vi "Update Waypoint Dictionary ConfigFile.vi"() -> ()   [LabVIEW 2020, in "WyPtDict.lvlib"]
uses:
  WyPtDict.lvlib
  RoboWaypointDict Node--cluster.ctl
  BRS_Dev/Source Code/Robo Driver/Controls/MC and Robo Handshake.ctl
  <vilib>/TELLC/Dynamic CVT API/TD Dynamic CVT DVR--ref.ctl
  <userlib>/_OpenG.lib/file/file.llb/File Exists - Scalar__ogtk.vi
panel:
  in  "Exit":bool
  in  "Save ConfigFile":bool
  in  "Load ConfigFile":bool
  in  "WyPtDictNode":T1[](array[typedef]) caption="Waypoint Configuration"
  in  "WaypointDictionary":T3
  in  "MainUI ViRef":refnum<vi>
  out "error out":errorcluster
  in  "error in (no error)":errorcluster
  out "Waypoint ConfigFile":path
  in  "WaypointDictionary":cluster{"WyPtDictNode":T1[]}
  # "XML Configuration File"
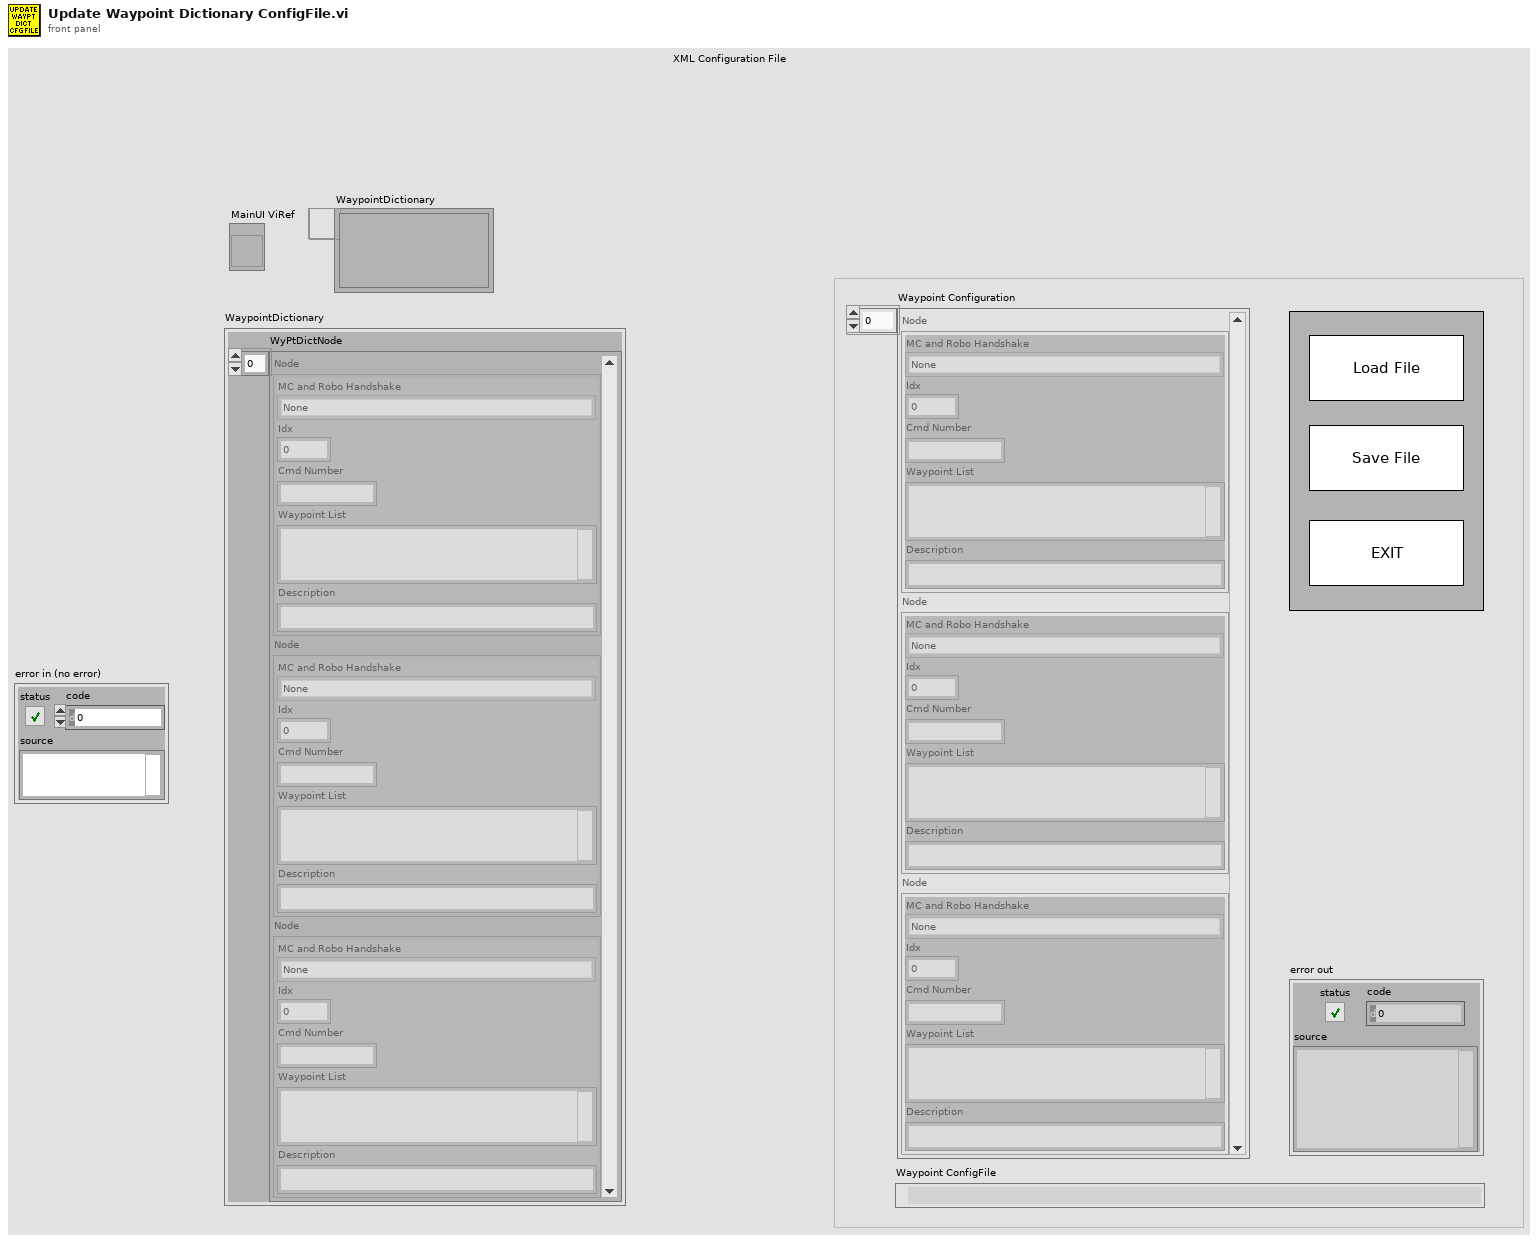
[diagram p1: front panel]
types:
  T1 = typedef "WyPtDict.lvlib/RoboWaypointDict Node--cluster.ctl" = cluster{"MC and Robo Handshake":T2, "Idx":i32, "Cmd Number":string, "Waypoint List":string, "Description":string}
  T2 = typedef "MC and Robo Handshake.ctl" = enum16{"None", "Move and Pick Nikon Ret LP(1100)", "Nikon Barcode1 Scanning Started(1101)", "Nikon Barcode1 Scan Abort(1102)", "Nikon Barcode1 Scan Success Proc to Barcode 2 Pos(1103)", "Nikon Barcode 2 Scanning Started(1104)", "Nikon Barcode 2 Scan Abort(1105) ", "Nikon Barcode 2 Success(1106)", "Move and Pick POZZ Ret LP(1300)", "POZZ Barcode Scan Started(1301)", "POZZ Barcode Not Found(1302)", "POZZ Barcode Scan Succ(1303)", "POZZ Mov to Side 2 Bar 2(1310)", "POZZ Mov to Side 4 Bar 1(1311)", "POZZ Mov to Side 4 Bar 2(1312)", "POZZ Mov to Side 1 Bar 1(1313)", "POZZ Mov to Side 1 Bar 2(1314)", "POZZ Mov to Side 3 Bar 1(1315)", "POZZ Mov to Side 3 Bar 2(1316)", "POZZ Mov to Edge 3 Nik 2(1317)", "POZZ Mov to Edge 4 ASML(1318)", "POZZ Mov to Edge 4 Nik 1(1319)", "POZZ Mov to Edge 4 Nik 2(1320)", "Move to ASML LP and Pick Ret(2000)", "ASML1 Barcode Scan Started(2001)", "ASML1 Barcode Not Found(2002)", "ASML1 Barcode Scan Succ(2003)", "Start Load Seq for Nikon LP(3000)", "Start Load Seq for POZZ LP(3200)", "Start Load Seq for ASML LP(3400)", "Start Align End Grip Place Func(4000)", "Start Align End grip Pick Func(4001)", "Start Align Center Grip Place Func(4002)", "Start Align Center grip Pick Func(4003)", "Start Move from home to Cleaner(5000)", "Start Move to Final Cleaner Loc(5001)", "Start Move from Cleaner loc to home(5002)", "Start Move from home to PDS for Inspect(6000) ", "PDS Inspect Finished(6001)", "PDS EMO Recovery(6002)", "Store in Stocker(7001)", "Store in Expansion Stocker(7401)", "Retrive from Center Stocker(8001)", "Retrive Mov to Nikon BC1 Scan Pos(8002)", "Retrive Nikon BC1not found(8003)", "Retrive Nikon BC1 Scan Succ(8004)", "Retrive Nikon BC2 not found(8005)", "Retrive Nikon BC2 scan Succ(8006)", "Retrive Mov to Edge 1 ASML(8202) ", "Retrive Mov to Edge 1 Nikon 1(8203)", "Retrive Mov to Edge 1 Nikon 2(8204)", "Retrive Mov to Edge 2 ASML(8205)", "Retrive Mov to Edge 2 Nikon 1(8206)", "Retrive Mov to Edge 2 Nikon 2(8207)", "Retrive Mov to Edge 3 ASML (8208)", "Retrive Mov to Edge 3 Nikon 1(8209)", "Retrive Mov to Edge 3 Nikon 2(8210)", "Retrive Mov to Edge 4 ASML (8211)", "Retrive Mov to Edge 4 Nikon 1 (8212)", "Retrive Mov to Edge 4 Nikon 2 (8213)", "Retrive BC Scan Abort (8214)", "Retrive BC Scan Successful (8215)", "Retrive Mov to ASML BC scan Pos (8402) ", "Retrive ASML BC not found(8403)", "Retrive ASML BC Scan Succ(8404)", "Expansion Retrive Seq (8601)", "Cen Stocker move from home to Transit Nest(9000)", "Cen Stocker move from Transit Nest to home(9200)", "Exp Stocker move from home to Transit Nest(9400)", "Exp Stocker move from Transit Nest to home(9600)", "Move to R1 Home (1000)", "Move to R2 Home (1000)", "Store Left Stocker (7401)", "Retrieve Left Stocker (8601)", "EMO Recovery Center (1002)", "EMO Recovery Right (1002)", "Center Robo Status (8888)", "Right Robo Status (8888)"}
  T3 = typedef "TD Dynamic CVT DVR--ref.ctl" = refnum<data-value>
  T4 = enum32{"Invalid", "Standard", "Closed", "Hidden", "Minimized", "Maximized"}
  T5 = cluster{"Core":cluster{"Current VI Reference":refnum<vi>, "Close Panel on Exit?":bool}, "WyPtDictNode":T1[], "ConfigFile":path}
  T6 = cluster{"Current VI Reference":refnum<vi>, "Close Panel on Exit?":bool}
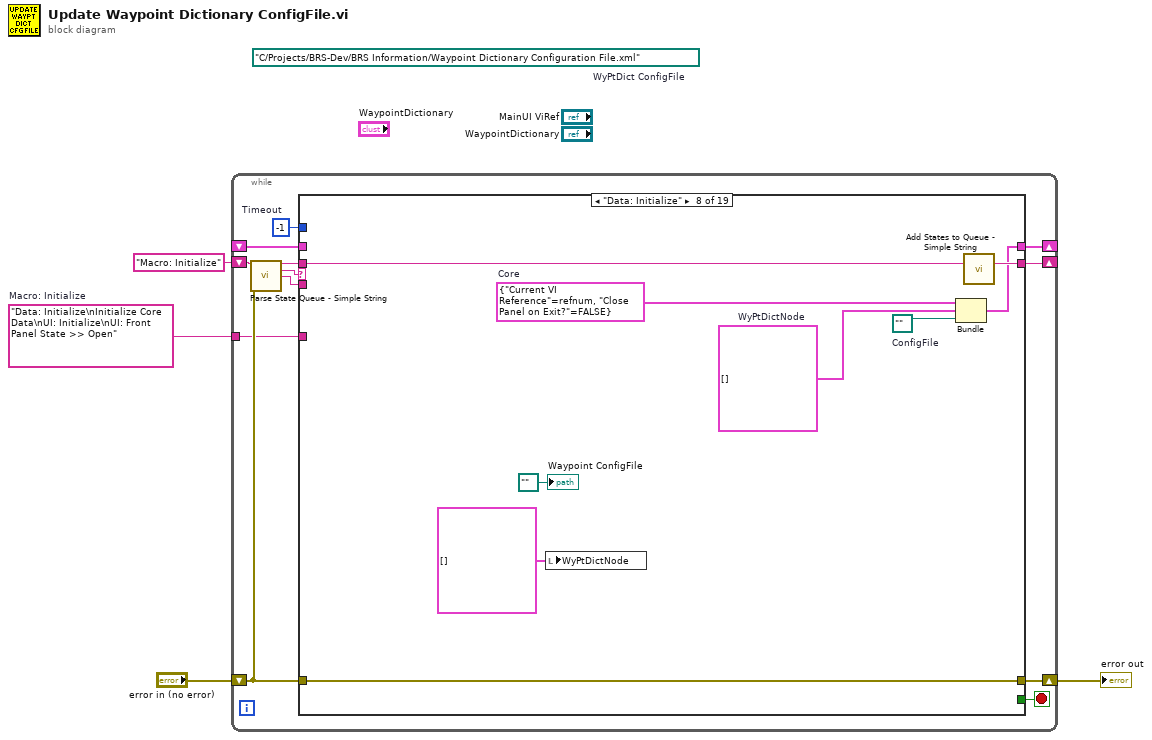
[diagram p0: block diagram]
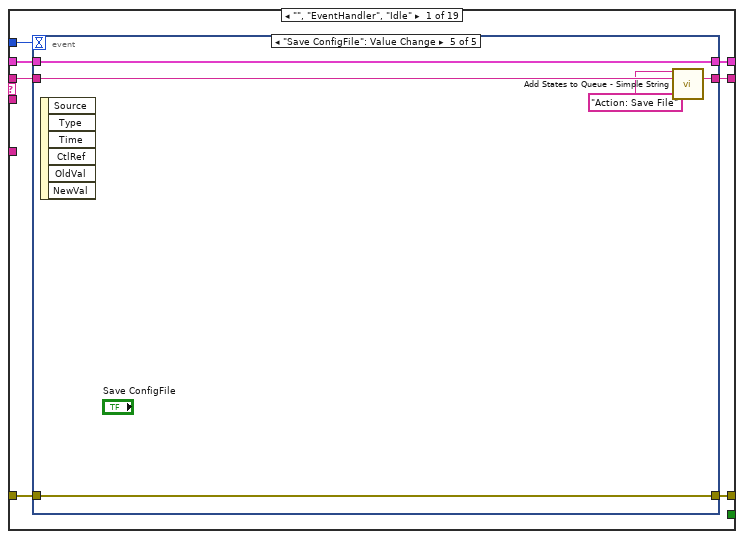
[diagram p2: hidden frame]
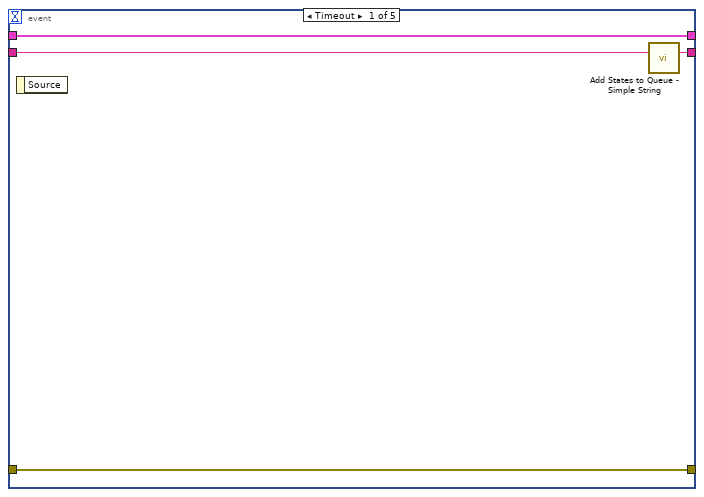
[diagram p3: hidden frame]
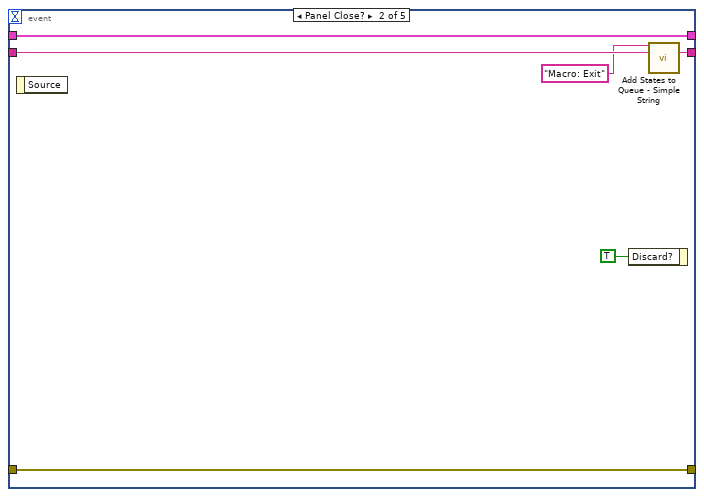
[diagram p4: hidden frame]
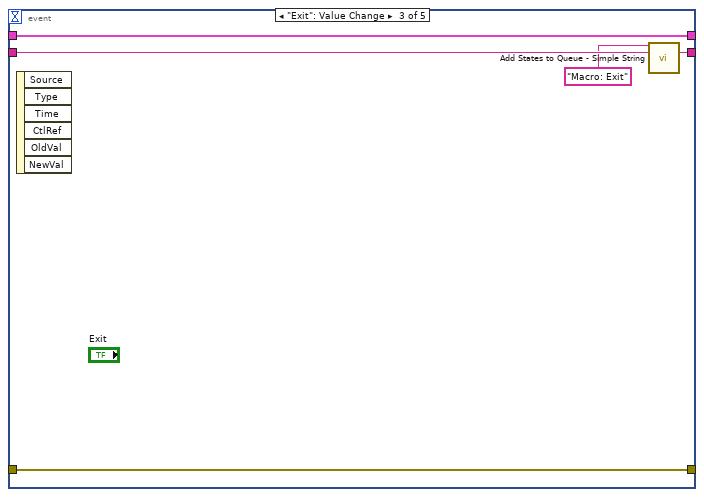
[diagram p5: hidden frame]
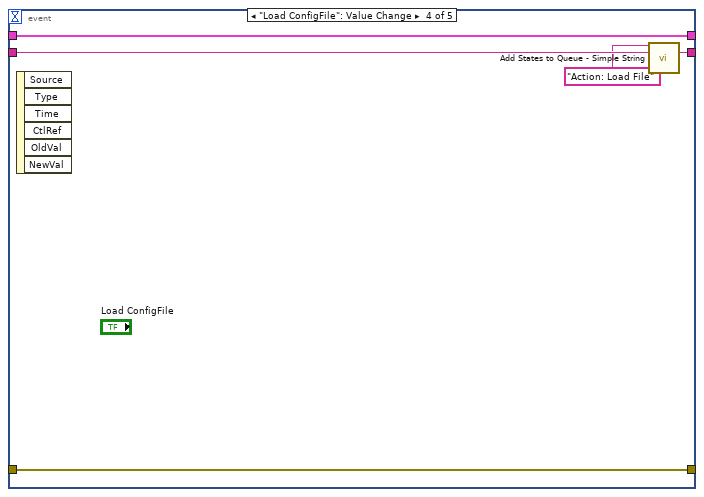
[diagram p6: hidden frame]
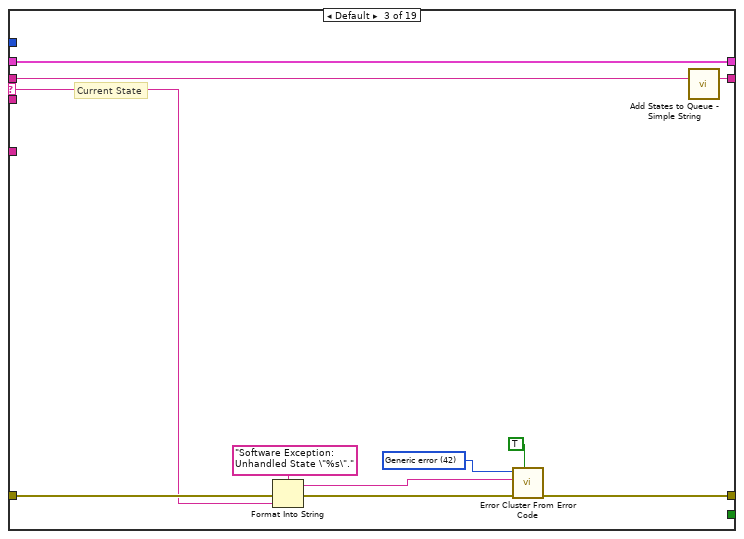
[diagram p8: hidden frame]
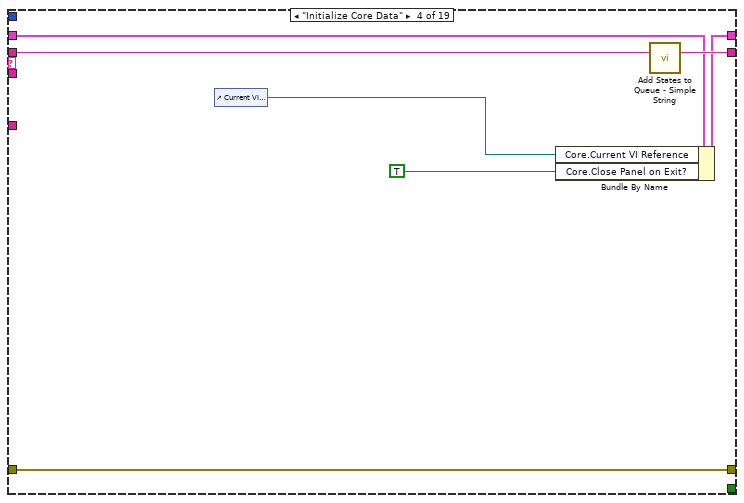
[diagram p9: hidden frame]
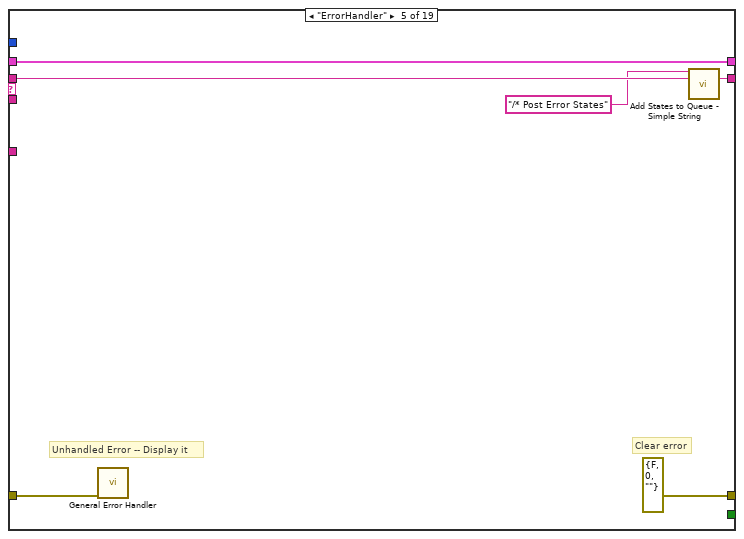
[diagram p10: hidden frame]
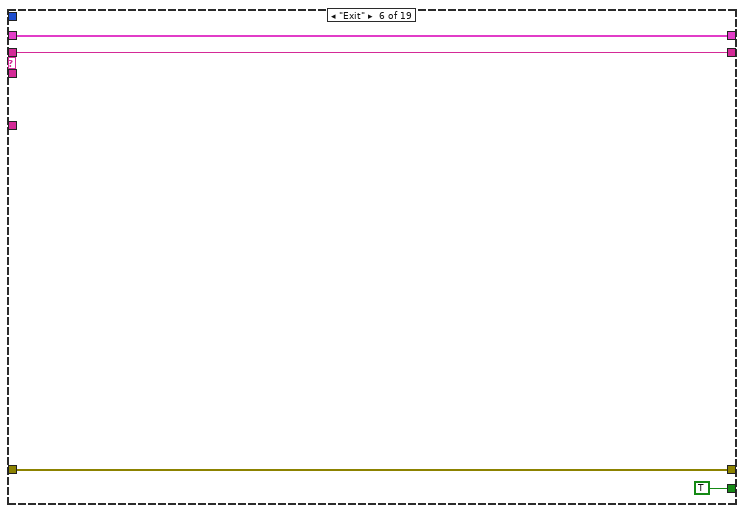
[diagram p11: hidden frame]
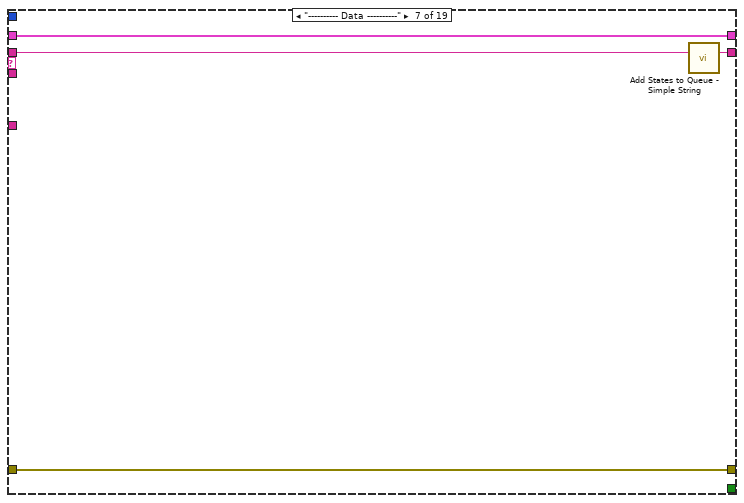
[diagram p12: hidden frame]
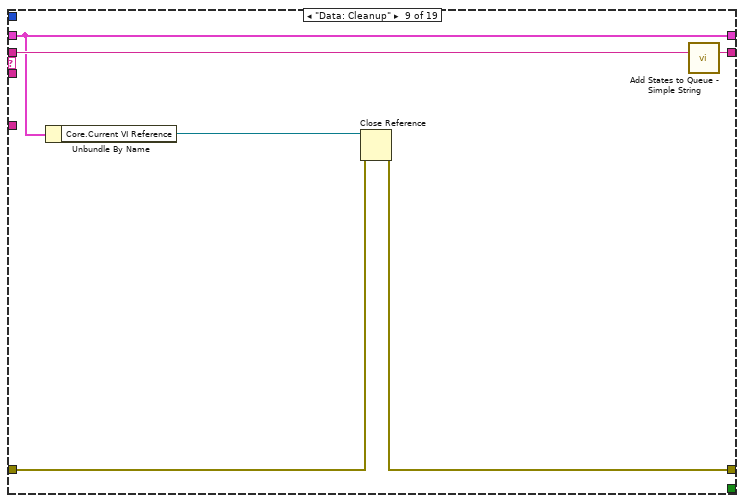
[diagram p13: hidden frame]
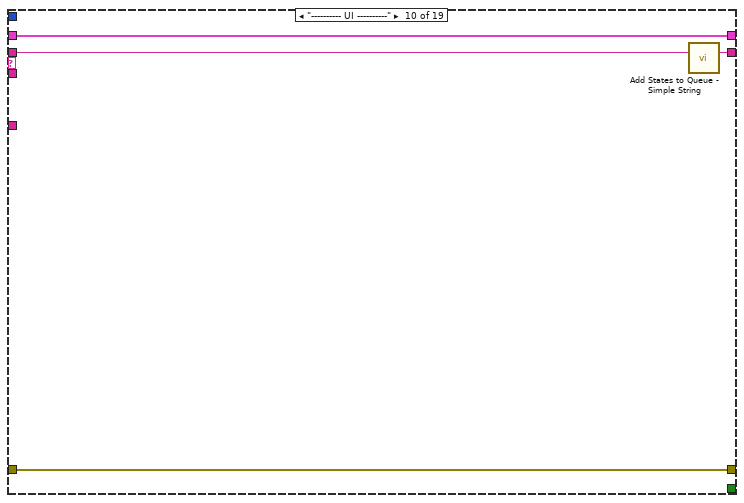
[diagram p14: hidden frame]
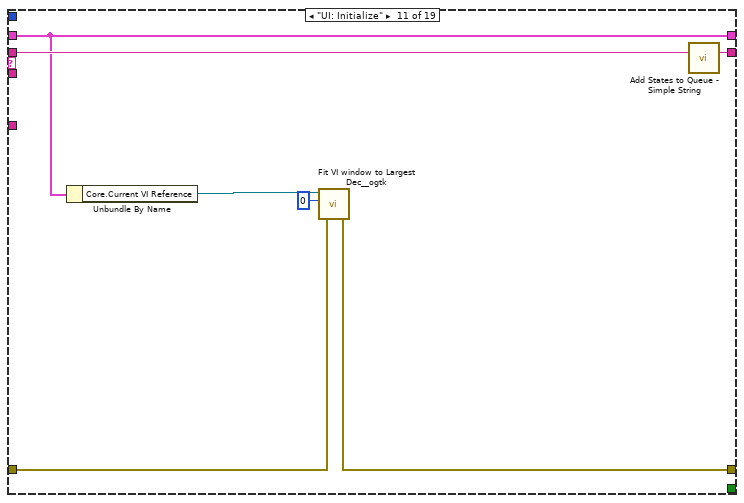
[diagram p15: hidden frame]
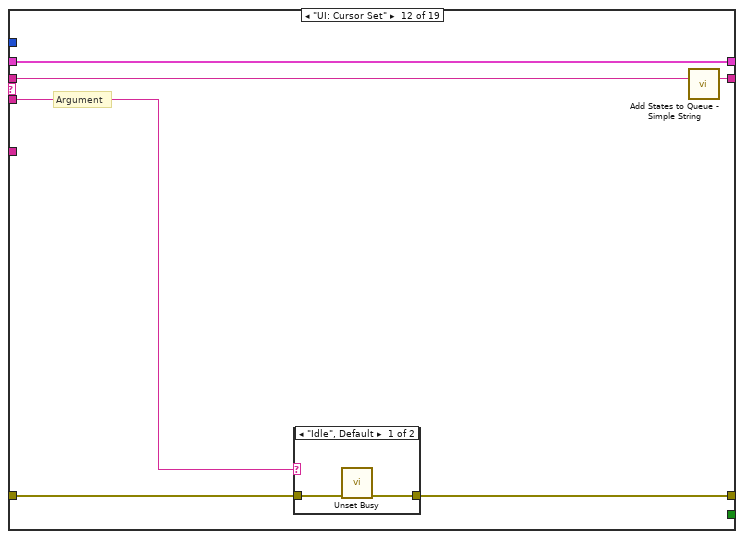
[diagram p16: hidden frame]
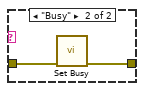
[diagram p17: hidden frame]
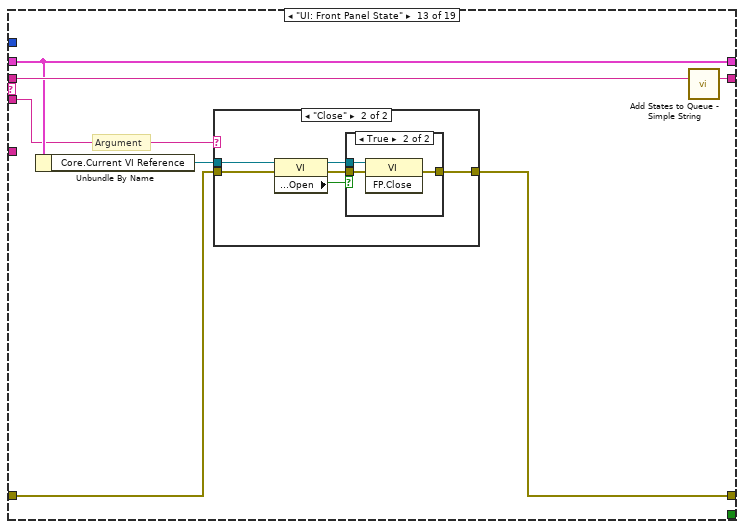
[diagram p18: hidden frame]
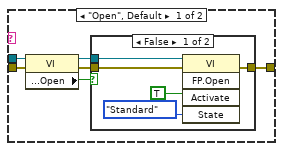
[diagram p19: hidden frame]
diagram:
  (unwired) path "C:/Projects/BRS-Dev/BRS Information/Waypoint Dictionary Configuration File.xml"  # WyPtDict ConfigFile
  w1 = "Data: Initialize\nInitialize Core Data\nUI: Initialize\nUI: Front Panel State >> Open"  # Macro: Initialize
  n1 = while {
    shift-right: [w9] -> _
    shift-left: _ -> [w8]
    shift-right: [w12] -> w3
    shift-left: "error in (no error)" -> [w6]
    shift-right: [w11] -> _
    shift-left: "Macro: Initialize" -> [w13]
    tunnel: w1 -> [w5]
    stop <- w10 stop-if-true
    w7 = -1  # Timeout
    n2 = call <vilib>:"Parse State Queue - Simple String.vi"("StateQ in"=w13, "error"=w6) -> ("Remaining States"=w15:string, "Next State"=w16:string, "Command (Optional)"=w14:string)  [unwired: 9 in, 2 out]
    n3 = case shown="\"Data: Initialize\"" w16 {
      selector: w16 -> [_ _ w52 _ _ _ _ _ _ _ _ _ _ _ _ _ _ _ _]
      tunnel: w15 -> [w23 w49 w56 w69 w75 w76 w83 w92 w98 w102 w109 w115 w126 w152 w157 w167 w171 w186 w208]
      tunnel: w14 -> [_ _ _ _ _ _ _ _ _ _ _ w110 w120 _ _ _ _ _ _]
      tunnel: w8 -> [w21 w50 w54 w65 w72 w79 w80 _ w93 w99 w107 w113 w122 w149 w154 w164 w168 w178 w203]
      tunnel: [w20 w51 w58 w66 errorcluster {"status"=FALSE, "code"=0, "source"=""} ("error out") w78 w81 w88 w94 w100 w104 w111 w123 w150 w155 w165 w169 w172 w199] -> w12
      tunnel: w6 -> [w19 w51 w57 w66 w71 w78 w81 w88 w95 w100 w103 w112 w124 w150 w155 w165 w169 w173 w200]
      tunnel: [w22 w49 w55 w68 w74 w76 w82 w91 w97 w101 w108 w114 w125 w151 w156 w166 w170 w185 w207] -> w11
      tunnel: [_ _ _ _ _ TRUE _ _ _ _ _ _ _ _ _ _ _ _ _] -> w10
      tunnel: [w18 w50 w54 w67 w72 w79 w80 w90 w93 w99 w107 w113 w122 w149 w154 w164 w168 w177 w202] -> w9
      tunnel: w7 -> [w17 _ _ _ _ _ _ _ _ _ _ _ _ _ _ _ _ _ _]
      tunnel: w5 -> [_ _ _ _ _ _ _ _ _ _ _ _ _ _ w153 _ _ _ _]
      frame "", "EventHandler", "Idle" {
        n4 = event shown="[4] \"Save ConfigFile\": Value Change" {
          selector: _ -> [_ _ _ _ _]
          dyn-events: _ -> [_ _ _ _ _]
          timeout: w17 -> [_ _ _ _ _]
          tunnel: w23 -> [w27 w33 w38 w43 w48]
          tunnel: [w26 w32 w37 w42 w47] -> w22
          tunnel: w21 -> [w24 w30 w35 w40 w45]
          tunnel: [w25 w31 w36 w41 w46] -> w20
          tunnel: w19 -> [w25 w31 w36 w41 w46]
          tunnel: [w24 w30 w35 w40 w45] -> w18
          event Timeout {
            n5 = event-data() -> ()  [unwired: 1 in, 1 out]
            n6 = call <vilib>:"Add States to Queue - Simple String.vi"("States in"=w27) -> ("States out"=w26:string)  [unwired: 14 in]
          }
          event Panel Close? {
            n7 = event-data() -> ()  [unwired: 1 in, 1 out]
            n8 = event-data("Discard?"=TRUE) -> ()  [unwired: 1 in, 1 out]
            n9 = call <vilib>:"Add States to Queue - Simple String.vi"("States in Front"="Macro: Exit", "States in"=w33) -> ("States out"=w32:string)  [unwired: 13 in]
          }
          event "Exit": Value Change {
            n10 = event-data() -> ()  [unwired: 1 in, 6 out]
            n11 = call <vilib>:"Add States to Queue - Simple String.vi"("States in Front"="Macro: Exit", "States in"=w38) -> ("States out"=w37:string)  [unwired: 13 in]
          }
          event "Load ConfigFile": Value Change {
            n12 = event-data() -> ()  [unwired: 1 in, 6 out]
            n13 = call <vilib>:"Add States to Queue - Simple String.vi"("States in Front"="Action: Load File", "States in"=w43) -> ("States out"=w42:string)  [unwired: 13 in]
          }
          event "Save ConfigFile": Value Change {
            n14 = event-data() -> ()  [unwired: 1 in, 6 out]
            n15 = call <vilib>:"Add States to Queue - Simple String.vi"("States in Front"="Action: Save File", "States in"=w48) -> ("States out"=w47:string)  [unwired: 13 in]
          }
        }
      }
      frame "---------- Core ----------" {
      }
      frame Default {
        w61 = 42 items=["No error", "Argument error", "Memory is full", "Out of zone", "End of file", "File already open", "Generic file I/O error", "File not found", "File permission error", "Disk is full", "Duplicate path", "Too many files open", "System feature not enabled", "Resource file not found", "Cannot add resource", "Resource not found", "Image not found", "Image memory error", "Pen does not exist", "Config type invalid", "Config token not found", "Config parse error", "Config memory error", "Bad external code format", "Bad external code offset", "External code not present", "Null window", "Destroy window error", "Null menu", "Print aborted", "Bad print record", "Print driver error", "Windows error during printing", "Memory error during printing", "Print dialog error", "Generic print error", "Invalid device refnum", "Device not found", "Device parameter error", "Device unit error", "Cannot open device", "Device call aborted", "Generic error", "Cancelled by user", "Object ID too low", "Object ID too high", "Object not in heap", "Unknown heap", "Unknown object (invalid DefProc)", "Unknown object (DefProc not in table)", "Message out of range", "Invalid (null) method", "Unknown message", "Manager call not supported", "Bad address", "Network operation in progress", "Network operation timed out", "Connection is busy", "Network attribute not supported", "Network error", "Address in use", "System out of memory", "Connection aborted", "Connection refused", "Not connected", "Already connected", "Connection closed", "Initialization error (interapplication manager)", "Bad occurrence", "Wait on unbound occurrence handler", "Occurrence queue overflow", "Datalog type conflict", "Unused", "Unrecognized type (interapplication manager)", "Memory corrupt", "Failed to make temporary DLL", "Old CIN version", "Drag socket not found", "Failed to load drop-object", "Failed to register OLE object", "Failed to release OLE object", "Format specifier type mismatch", "Unknown format specifier", "Too few format specifiers", "Too many format specifiers", "Scan failed", "Newer CIN version", "Error converting to variant", "Runtime menu error", "Password tampered", "Variant attribute not found", "Incompatible variant data type", "Event data is not available", "Event Store is not present", "Occurrence is not found", "Event Queue is not created", "Event info is not available", "Refnum passed is NULL", "Error retrieving Class GUID", "Error retrieving CoClass GUID", "Error retrieving TypeLib GUID.", "Bad built application magic bytes.", "Specific driver is different from the specific driver associated with the Logical Name.", "There is no session opened to the class driver.", "Max Error", "MAX - Error with config objects", "MAX - Error loading configuration", "MAX - Group not supported"]
        # "Current State"
        n16 = Format Into String(format string="Software Exception: Unhandled State \"%s\"." ("message"), error in=w57, w52) -> (resulting string=w60:string, error out=w59:errorcluster)  [unwired: 1 in]
        n17 = call <vilib>:"Error Cluster From Error Code.vi"("show call chain? (False)"=TRUE, "error in (no error)"=w59, "error message (\"\")"=w60, "error code (0)"=w61) -> ("error out"=w58:errorcluster)  [unwired: 5 in]
        n18 = call <vilib>:"Add States to Queue - Simple String.vi"("States in"=w56) -> ("States out"=w55:string)  [unwired: 14 in]
      }
      frame "Initialize Core Data" {
        n19 = control-ref of="Current VI Reference"() -> (w64:refnum<vi>)
        n20 = Bundle By Name(cluster=w65, "Core.Current VI Reference"=w64, "Core.Close Panel on Exit?"=TRUE) -> (w67:T5)
        n21 = call <vilib>:"Add States to Queue - Simple String.vi"("States in"=w69) -> ("States out"=w68:string)  [unwired: 14 in]
      }
      frame "ErrorHandler" {
        # "Unhandled Error -- Display it"
        # "Clear error"
        n22 = call <vilib>:"General Error Handler.vi"("error in (no error)"=w71) -> ()  [unwired: 10 in, 5 out]
        n23 = call <vilib>:"Add States to Queue - Simple String.vi"("States in Front"="/* Post Error States", "States in"=w75) -> ("States out"=w74:string)  [unwired: 13 in]
      }
      frame "Exit" {
      }
      frame "---------- Data ----------" {
        n24 = call <vilib>:"Add States to Queue - Simple String.vi"("States in"=w83) -> ("States out"=w82:string)  [unwired: 14 in]
      }
      frame "Data: Initialize" {
        w86 = path ""  # ConfigFile
        w87 = T1[] []  # WyPtDictNode
        w89 = T6 {"Current VI Reference"=refnum, "Close Panel on Exit?"=FALSE}  # Core
        n25 = local write "WyPtDictNode"(T1[] [] ("WyPtDictNode")) -> ()
        n26 = Bundle("Core"=w89, "WyPtDictNode"=w87, "ConfigFile"=w86) -> (w90:T5)  [unwired: 1 in]
        n27 = call <vilib>:"Add States to Queue - Simple String.vi"("States in"=w92) -> ("States out"=w91:string)  [unwired: 14 in]
        "Waypoint ConfigFile" <- path "" ("Waypoint ConfigFile")
      }
      frame "Data: Cleanup" {
        n28 = Unbundle By Name(w93) -> ("Core.Current VI Reference"=w96:refnum<vi>)
        n29 = Close Reference(reference=w96, error in (no error)=w95) -> (error out=w94:errorcluster)
        n30 = call <vilib>:"Add States to Queue - Simple String.vi"("States in"=w98) -> ("States out"=w97:string)  [unwired: 14 in]
      }
      frame "---------- UI ----------" {
        n31 = call <vilib>:"Add States to Queue - Simple String.vi"("States in"=w102) -> ("States out"=w101:string)  [unwired: 14 in]
      }
      frame "UI: Initialize" {
        n32 = Unbundle By Name(w107) -> ("Core.Current VI Reference"=w106:refnum<vi>)
        n33 = call <userlib>:"Fit VI window to Largest Dec__ogtk.vi"("error in (no error)"=w103, "border spacing (2 px)"=0, "VI Ref (calling VI)"=w106) -> ("error out"=w104:errorcluster)  [unwired: 3 in, 1 out]
        n34 = call <vilib>:"Add States to Queue - Simple String.vi"("States in"=w109) -> ("States out"=w108:string)  [unwired: 14 in]
      }
      frame "UI: Cursor Set" {
        # "Argument"
        n35 = case shown="\"Idle\", Default" w110 {
          tunnel: w112 -> [w117 w119]
          tunnel: [w116 w118] -> w111
          frame "Idle", Default {
            n36 = call <vilib>:"Unset Busy.vi"("error in (no error)"=w117) -> ("error out"=w116:errorcluster)  [unwired: 10 in]
          }
          frame "Busy" {
            n37 = call <vilib>:"Set Busy.vi"("error in (no error)"=w119) -> ("error out"=w118:errorcluster)  [unwired: 9 in, 1 out]
          }
        }
        n38 = call <vilib>:"Add States to Queue - Simple String.vi"("States in"=w115) -> ("States out"=w114:string)  [unwired: 14 in]
      }
      frame "UI: Front Panel State" {
        # "Argument"
        n39 = Unbundle By Name(w122) -> ("Core.Current VI Reference"=w121:refnum<vi>)
        n40 = case shown="\"Close\"" w120 {
          tunnel: w124 -> [w130 w143]
          tunnel: [w132 w144] -> w123
          tunnel: w121 -> [w131 w141]
          frame "Open", Default {
            n41 = property class="VI"(reference=w131, error in=w130) -> (reference out=w128:refnum<vi>, error out=w129:errorcluster, "Front Panel.Open"=w127:bool)
            n42 = case shown="False" w127 {
              tunnel: [w135 w138] -> w132
              tunnel: w129 -> [w134 w138]
              tunnel: w128 -> [w133 _]
              frame False {
                n43 = invoke class="VI" method="FP.Open"(reference=w133, error in=w134, "Activate"=TRUE, "State"=T4."Standard") -> (error out=w135:errorcluster)  [unwired: 1 in, 4 out]
              }
              frame True {
              }
            }
          }
          frame "Close" {
            n44 = property class="VI"(reference=w141, error in=w143) -> (reference out=w140:refnum<vi>, error out=w142:errorcluster, "Front Panel.Open"=w139:bool)
            n45 = case shown="True" w139 {
              tunnel: [w145 w148] -> w144
              tunnel: w142 -> [w145 w147]
              tunnel: w140 -> [_ w146]
              frame False {
              }
              frame True {
                n46 = invoke class="VI" method="FP.Close"(reference=w146, error in=w147) -> (error out=w148:errorcluster)  [unwired: 1 in, 2 out]
              }
            }
          }
        }
        n47 = call <vilib>:"Add States to Queue - Simple String.vi"("States in"=w126) -> ("States out"=w125:string)  [unwired: 14 in]
      }
      frame "---------- Macro ----------" {
        n48 = call <vilib>:"Add States to Queue - Simple String.vi"("States in"=w152) -> ("States out"=w151:string)  [unwired: 14 in]
      }
      frame "Macro: Initialize" {
        n49 = call <vilib>:"Add States to Queue - Simple String.vi"("States in Front"=w153, "States in"=w157) -> ("States out"=w156:string)  [unwired: 13 in]
      }
      frame "Macro: Exit" {
        n50 = Unbundle By Name(w164) -> ("Core.Close Panel on Exit?"=w163:bool)
        n51 = Select(t="UI: Front Panel State >> Close", s=w163, f="") -> (s? t:f=w160:string)
        n52 = call <vilib>:"Add States to Queue - Simple String.vi"("States in"=w160, "States at Back"="Data: Cleanup\nExit") -> ("States out"=w158:string)  [unwired: 13 in]
        n53 = call <vilib>:"Add States to Queue - Simple String.vi"("States in Front"=w158, "States in"=w167) -> ("States out"=w166:string)  [unwired: 13 in]
      }
      frame "---------- Action ----------" {
        n54 = call <vilib>:"Add States to Queue - Simple String.vi"("States in"=w171) -> ("States out"=w170:string)  [unwired: 14 in]
      }
      frame "Action: Load File" {
        n55 = Unbundle By Name(w178) -> ("ConfigFile"=w184:path)
        n56 = call "File Dialog"("start path"=w184, "prompt"="Select Waypoint Configuration File to Load (XML)", "button label"="Open", "error in"=w173, "pattern (all files)"="*.xml") -> ("selected path"=w180:path, "exists"=w175:bool, "cancelled"=w176:bool, "error out"=w179:errorcluster)  [unwired: 7 in]
        n57 = Compound Arithmetic op=AND(w175, invert w176) -> (w174:bool)
        n58 = case shown="True" w174 {
          tunnel: w180 -> [_ w196]
          tunnel: w179 -> [w187 w195]
          tunnel: w178 -> [w188 w193]
          tunnel: [w188 w192] -> w177
          tunnel: [w187 w190] -> w172
          frame False {
          }
          frame True {
            n59 = call "Read Waypoint Dictionary ConfigFile.vi"("error in (no error)"=w195, "Waypoint Dictionary ConfigFile"=w196) -> ("error out"=w190:errorcluster, "WaypointDictionary"=w194:cluster{"WyPtDictNode":T1[]}, "Path"=w189:path)  [unwired: 7 in]
            n60 = local write "Waypoint ConfigFile"(w189) -> ()
            n61 = Unbundle(w194) -> ("WyPtDictNode"=w191:T1[])
            n62 = local write "WyPtDictNode"(w191) -> ()
            n63 = Bundle By Name(cluster=w193, "ConfigFile"=w189) -> (w192:T5)
          }
        }
        n64 = call <vilib>:"Add States to Queue - Simple String.vi"("States in"=w186) -> ("States out"=w185:string)  [unwired: 14 in]
      }
      frame "Action: Save File" {
        n65 = Unbundle By Name(w203) -> ("ConfigFile"=w198:path)
        n66 = call-poly <userlib>:"File Exists__ogtk.vi"("file path"=w198) -> ("exists"=w197:bool)  [unwired: 6 in, 1 out]
        n67 = case shown="False" w197 {
          tunnel: "Select Waypoint Configuration File to Save (XML)" ("prompt") -> [w217 _]
          tunnel: [w215 w221] -> w205
          tunnel: [w214 w220] -> w204
          tunnel: [w211 TRUE] -> w201
          tunnel: w200 -> [w210 w220]
          tunnel: w198 -> [w209 w221]
          frame False {
            n68 = call "File Dialog2"("start path"=w209, "prompt"=w217, "button label"="Save", "error in"=w210, "pattern (all files)"="*.xml") -> ("selected path"=w215:path, "exists"=w212:bool, "cancelled"=w213:bool, "error out"=w214:errorcluster)  [unwired: 7 in]
            n69 = Compound Arithmetic op=AND(w212, invert w213) -> (w211:bool)
          }
          frame True {
          }
        }
        n70 = case shown="True" w201 {
          tunnel: w205 -> [_ w227]
          tunnel: w204 -> [w222 w229]
          tunnel: w203 -> [w223 w231]
          tunnel: [w223 w230] -> w202
          tunnel: [w222 w228] -> w199
          frame False {
          }
          frame True {
            n71 = Bundle("WyPtDictNode"="WyPtDictNode") -> (w225:cluster{"WyPtDictNode":T1[]})  [unwired: 1 in]
            n72 = call "Write Waypoint Dictionary ConfigFile.vi"("error in (no error)"=w229, "WaypointDictionary"=w225, "Waypoint Dictionary ConfigFile"=w227) -> ("error out"=w228:errorcluster, "XML File Path (duplicate)"=w224:path)  [unwired: 7 in]
            n73 = local write "Waypoint ConfigFile"(w224) -> ()
            n74 = Bundle By Name(cluster=w231, "ConfigFile"=w224) -> (w230:T5)
          }
        }
        n75 = call <vilib>:"Add States to Queue - Simple String.vi"("States in"=w208) -> ("States out"=w207:string)  [unwired: 14 in]
      }
    }
  }
  "error out" <- w3
